vi "Remove Logging Library Callers.vi"(11 "call chain":string[](array[string])) -> (3 "trimmed call chain":string[](array[string]))   [LabVIEW 2018, in "GLog.lvlib" / "Scope.lvclass"]
uses:
  extension/scope_interface/Scope.lvclass
panel:
  # "Connector Pane"
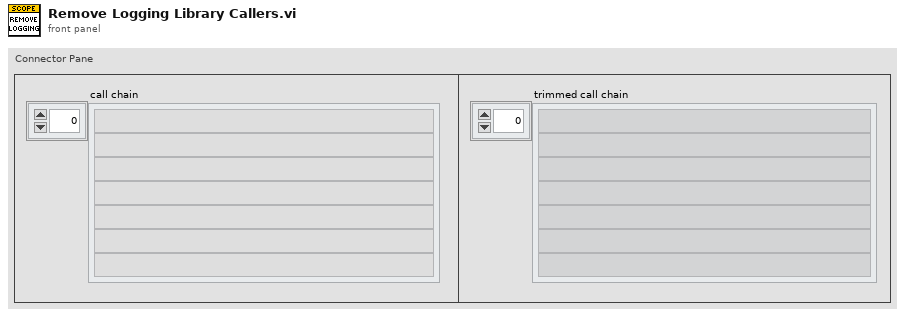
[diagram p1: front panel]
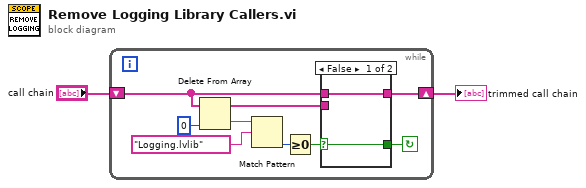
[diagram p0: block diagram]
diagram:
  n1 = while {
    shift-right: [w4] -> w1
    shift-left: "call chain" -> [w7]
    stop <- w5 continue-if-true
    n2 = Delete From Array(array=w7, index=0) -> (deleted portion=w6:string, array with subset deleted=w8:string[])  [unwired: 1 in]
    n3 = Match Pattern(string=w6, regular expression="Logging.lvlib") -> (offset past match=w10:i32)  [unwired: 1 in, 3 out]
    n4 = Greater Or Equal To 0?(x=w10) -> (x >= 0?=w9:bool)
    n5 = case shown="False" w9 {
      selector: w9 -> [w12 w15]
      tunnel: w8 -> [_ w14]
      tunnel: [w12 w15] -> w5
      tunnel: w7 -> [w13 _]
      tunnel: [w13 w14] -> w4
      frame False {
      }
      frame True {
      }
    }
  }
  "trimmed call chain" <- w1
